vi "SaveTestFile.vi"(8 "ErrorArray In":errorcluster[](array[cluster])) -> (0 "ErrorArray Out":errorcluster[](array[cluster]))   [LabVIEW 2014, in "Framework.lvlib"]
uses:
  Framework.lvlib
  Config_class/Config.lvclass/Config.ctl
  Config_class/Accessors/Read PARTF Root Directory.vi
  <userlib>/NIST/NISTErrorLib/NISTErrorLib.lvlib
  Bus_class/Bus.lvclass
  <vilib>/Utility/config.llb/NI_LVConfig.lvlib
  Config_class/Config.lvclass
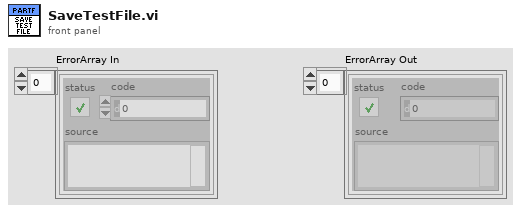
[diagram p1: front panel]
types:
  T1 = typedef "Framework.lvlib/clFrontPanelControlRefs.ctl" = cluster{"TestFilePathRef":refnum<vi>, "BusNumberRef":refnum<vi>, "NumberOfBusesRef":refnum<vi>, "EvtTypeRef":refnum<vi>, "EvtParamsRef":refnum<vi>, "EvtConfigRef":refnum<vi>, "StartTimeRef":refnum<vi>, "EndTimeRef":refnum<vi>, "PmuImpairTypeRef":refnum<vi>, "PmuImpairParamsRef":refnum<vi>, "NetImpairParamsRef":refnum<vi>, "FlagImpairTypeRef":refnum<vi>, "FlagImpairParamsRef":refnum<vi>, "NetImpairTypeRef":refnum<vi>, "OutputFileType":refnum<vi>, "PmuImpairConfigRef":refnum<vi>, "AppTypeRef":refnum<vi>, "ScriptPathRef":refnum<vi>, "ShowPanels?":refnum<vi>}
  T2 = typedef "Framework.lvlib/Config.lvclass/RootDir.ctl" = cluster{"pathRootDir":path, "btnOutPath":bool, "OutDir":string, "btnOpenOutputDir":bool, "ScriptDir":string, "btnOpenScriptDir":bool, "TestDir":string, "btnOpenTestDir":bool}
  T3 = typedef "Framework.lvlib/clFrameworkData.ctl" = cluster{"EvtINIFilePaths":path[], "BusClassInstances":refnum<class "Bus.lvclass">[], "PmuImpairINIFilePaths":path[], "FlagImpairINIFilePaths":path[], "NetImpairINIFilePaths":path[], "OutputToFileINIFilePaths":path[], "AppINIFilePaths":path[], "AppModuleID":i32, "OutputToFileID":i32}
  T4 = typedef "NI_LVConfig.lvlib/Config Data RefNum.ctl" = refnum<k1>
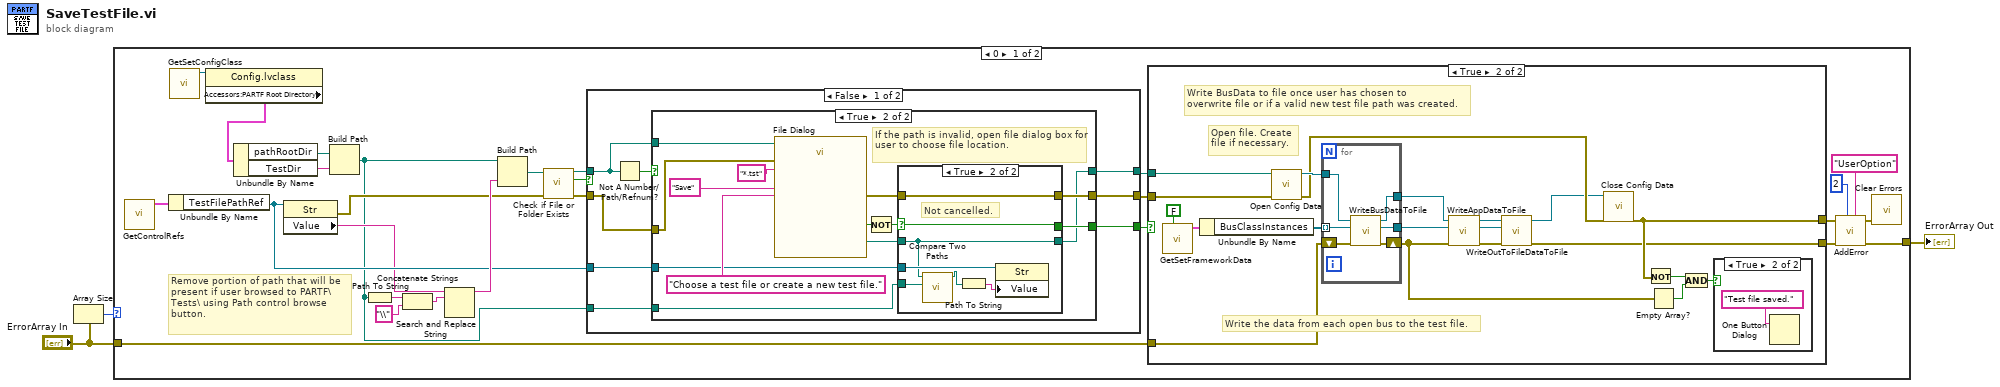
[diagram p0: block diagram]
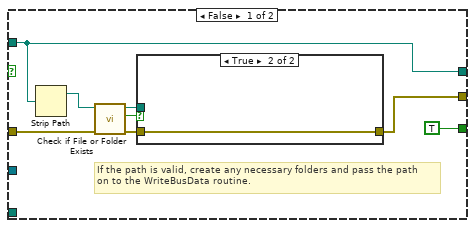
[diagram p4: hidden frame]
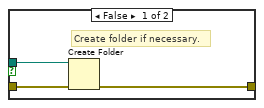
[diagram p5: hidden frame]
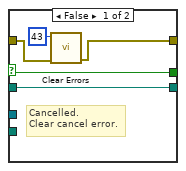
[diagram p6: hidden frame]
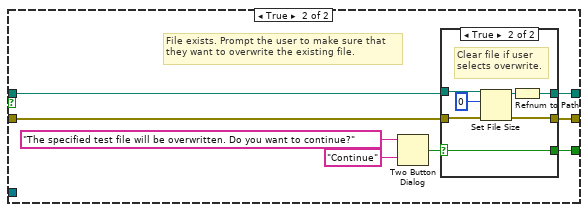
[diagram p7: hidden frame]
diagram:
  n1 = Array Size(array="ErrorArray In") -> (size(s)=w3:i32)
  n2 = case shown="0" w3 {
    tunnel: "ErrorArray In" -> [w26 w124]
    tunnel: [w11 w124] -> w1
    frame 0 {
      # "Remove portion of path that will be present if user browsed to PARTF\\Tests\\ using Path control browse button."
      n3 = call "GetControlRefs.vi"() -> ("clControlRefs Out"=w6:T1)  [unwired: 11 in]
      n4 = Unbundle By Name(w6) -> ("TestFilePathRef"=w13:refnum<vi>)
      n5 = call "GetSetConfigClass.vi"() -> ("Ref out"=w10:refnum<class "Config.lvclass">)  [unwired: 11 in]
      n6 = property class="Config.lvclass"(reference=w10) -> ("Accessors:PARTF Root Directory"=w9:T2)  [unwired: 1 in, 2 out]
      n7 = Unbundle By Name(w9) -> ("pathRootDir"=w8:path, "TestDir"=w7:string)
      n8 = property class="Str"(reference=w13) -> (error out=w20:errorcluster, "Value"=w5:string)  [unwired: 1 in, 1 out]
      n9 = Build Path(base path=w8, name or relative path=w7) -> (appended path=w4:path)
      n10 = Path To String(path=w4) -> (string=w25:string)
      n11 = Concatenate Strings(w25, "\\" ("string")) -> (w23:string)
      n12 = Search and Replace String(input string=w5, search string=w23) -> (result string=w24:string)  [unwired: 6 in, 3 out]
      n13 = Build Path(base path=w4, name or relative path=w24) -> (appended path=w21:path)
      n14 = call <vilib>:"Check if File or Folder Exists.vi"("error in (no error)"=w20, "path"=w21) -> ("error out"=w17:errorcluster, "file or folder exists?"=w19:bool, "dup path"=w18:path)  [unwired: 7 in]
      n15 = case shown="False" w19 {
        tunnel: w18 -> [w65 w113]
        tunnel: w17 -> [w66 w112]
        tunnel: [w67 w110] -> w16
        tunnel: [w63 w111] -> w15
        tunnel: [w61 w106] -> w14
        tunnel: w13 -> [w62 _]
        tunnel: w4 -> [w60 _]
        frame False {
          n16 = Not A Number/Path/Refnum?(number/path/refnum=w65) -> (NaN/Path/Refnum?=w64:bool)
          n17 = case shown="True" w64 {
            tunnel: [w75 w86] -> w67
            tunnel: w65 -> [w69 w93]
            tunnel: w66 -> [w71 w92]
            tunnel: [w69 w81] -> w63
            tunnel: w62 -> [_ w84]
            tunnel: [TRUE w83] -> w61
            tunnel: w60 -> [_ w80]
            frame False {
              # "If the path is valid, create any necessary folders and pass the path\non to the WriteBusData routine."
              n18 = Strip Path(path=w69) -> (stripped path=w73:path)  [unwired: 1 out]
              n19 = call <vilib>:"Check if File or Folder Exists.vi"("error in (no error)"=w71, "path"=w73) -> ("error out"=w72:errorcluster, "file or folder exists?"=w74:bool, "dup path"=w70:path)  [unwired: 7 in]
              n20 = case shown="True" w74 {
                tunnel: w72 -> [w77 w79]
                tunnel: [w78 w79] -> w75
                tunnel: w70 -> [w76 _]
                frame False {
                  # "Create folder if necessary."
                  n21 = Create Folder(path (use dialog)=w76, error in=w77) -> (error out=w78:errorcluster)  [unwired: 1 in, 2 out]
                }
                frame True {
                }
              }
            }
            frame True {
              # "If the path is invalid, open file dialog box for user to choose file location."
              n22 = call "File Dialog"("start path"=w93, "prompt"="Choose a test file or create a new test file.", "button label"="Save", "error in"=w92, "pattern (all files)"="*.tst") -> ("selected path"=w85:path, "cancelled"=w88:bool, "error out"=w87:errorcluster)  [unwired: 7 in, 1 out]
              n23 = Not(x=w88) -> (.not. x?=w82:bool)
              n24 = case shown="True" w82 {
                selector: w82 -> [w95 w104]
                tunnel: w87 -> [w98 w105]
                tunnel: [w97 w105] -> w86
                tunnel: [w95 w104] -> w83
                tunnel: w85 -> [w94 w102]
                tunnel: w84 -> [_ w103]
                tunnel: [w94 w102] -> w81
                tunnel: w80 -> [_ w101]
                frame False {
                  # "Cancelled.\nClear cancel error."
                  n25 = call <vilib>:"Clear Errors.vi"("error in (no error)"=w98, "specific error code to clear (0: all)"=43) -> ("error out"=w97:errorcluster)  [unwired: 4 in, 1 out]
                }
                frame True {
                  # "Not cancelled."
                  n26 = call <vilib>:"Compare Two Paths.vi"("Path 2"=w101, "Path 1"=w102) -> ("Relative Path from 1 to 2"=w99:path)  [unwired: 6 in, 3 out]
                  n27 = Path To String(path=w99) -> (string=w100:string)
                  n28 = property class="Str"(reference=w103, "Value"=w100) -> ()  [unwired: 1 in, 2 out]
                }
              }
            }
          }
        }
        frame True {
          # "File exists. Prompt the user to make sure that\nthey want to overwrite the existing file."
          n29 = Two Button Dialog(message="The specified test file will be overwritten. Do you want to continue?", 2:"Continue" ("T button name (\"OK\")")) -> (T button?=w109:bool)  [unwired: 1 in]
          n30 = case shown="True" w109 {
            selector: w109 -> [w116 w117]
            tunnel: w113 -> [w114 w122]
            tunnel: w112 -> [w115 w121]
            tunnel: [w114 w119] -> w111
            tunnel: [w115 w118] -> w110
            tunnel: [w116 w117] -> w106
            frame False {
            }
            frame True {
              # "Clear file if user\nselects overwrite."
              n31 = Set File Size(4:w121, 6:i64 0 ("size (in bytes)"), 7:w122) -> (0:w118:errorcluster, 3:w120:refnum<file>)
              n32 = Refnum to Path(1:w120) -> (0:w119:path)
            }
          }
        }
      }
      n33 = case shown="True" w14 {
        tunnel: [w32 w43] -> w27
        tunnel: w26 -> [w31 w52]
        tunnel: [w31 w36] -> w12
        tunnel: w16 -> [w32 w46]
        tunnel: w15 -> [_ w45]
        frame False {
          # "Don't save file.  User cancelled."
        }
        frame True {
          # "Write BusData to file once user has chosen to \noverwrite file or if a valid new test file path was created."
          # "Write the data from each open bus to the test file."
          # "Open file. Create\nfile if necessary."
          n34 = call "GetSetFrameworkData.vi"("Set (F)"=FALSE ("Set/Get")) -> ("clFrameworkData Out"=w50:T3)  [unwired: 10 in]
          n35 = Unbundle By Name(w50) -> ("BusClassInstances"=w47:refnum<class "Bus.lvclass">[])
          n36 = call <vilib>:"Open Config Data.vi"("error in (no error)"=w46, "configuration file path"=w45) -> ("error out"=w48:errorcluster, "refnum"=w49:T4)  [unwired: 7 in, 1 out]
          n37 = for {
            tunnel: w49 -> [w56]
            tunnel: w47 -> [w57] mode=indexing
            shift-right: [w59] -> w40
            shift-left: w52 -> [w55]
            tunnel: [w58] -> w39
            tunnel: [w54] -> w38
            n38 = call "WriteBusDataToFile.vi"("ErrorArray In"=w55, "Bus.lvclass In"=w57, "TestFileRef In"=w56) -> ("ErrorArray Out"=w59:errorcluster[], "Bus.lvclass Out"=w54:refnum<class "Bus.lvclass">, "TestFileRef Out"=w58:T4)  [unwired: 6 in]
          }
          n39 = call "WriteAppDataToFile.vi"("ErrorArray In"=w40, "Bus.lvclass In"=w38, "TestFileRef In"=w39) -> ("ErrorArray Out"=w37:errorcluster[], "Bus.lvclass Out"=w33:refnum<class "Bus.lvclass">, "TestFileRef Out"=w35:T4)  [unwired: 6 in]
          n40 = call "WriteOutToFileDataToFile.vi"("ErrorArray In"=w37, "Bus.lvclass In"=w33, "TestFileRef In"=w35) -> ("ErrorArray Out"=w36:errorcluster[], "TestFileRef Out"=w34:T4)  [unwired: 6 in, 1 out]
          n41 = call <vilib>:"Close Config Data.vi"("error in (no error)"=w48, "refnum"=w34) -> ("error out"=w43:errorcluster)  [unwired: 8 in, 1 out]
          n42 = Not(x=w43) -> (.not. x?=w42:bool)
          n43 = Empty Array?(array=w40) -> (empty?=w41:bool)
          n44 = And(x=w42, y=w41) -> (x .and. y?=w44:bool)
          n45 = case shown="True" w44 {
            frame False {
            }
            frame True {
              n46 = One Button Dialog(message="Test file saved.") -> ()  [unwired: 1 in, 1 out]
            }
          }
        }
      }
      n47 = call <userlib>:"AddError.vi"("Severity"="UserOption" ("String"), "Priority"=u8 2, "ErrorArray"=w12, "error in (no error)"=w27) -> ("ErrorArray"=w11:errorcluster[], "error out"=w30:errorcluster)  [unwired: 6 in]
      n48 = call <vilib>:"Clear Errors.vi"("error in (no error)"=w30) -> ()  [unwired: 5 in, 2 out]
    }
    frame 1, Default {
    }
  }
  "ErrorArray Out" <- w1
